vi "target.vi"   [LabVIEW 2020]
uses:
  <vilib>/rvi/interface/RandomDataEmulation/niFpgaRandomDataHandleErrors.vi
  <vilib>/rvi/DataTransferAndStorage/Container/XNode/niFpgaContainer.xnode
  <vilib>/rvi/interface/RandomDataEmulation/nirviRandomDataFpgaReadWriteTemplate.vi
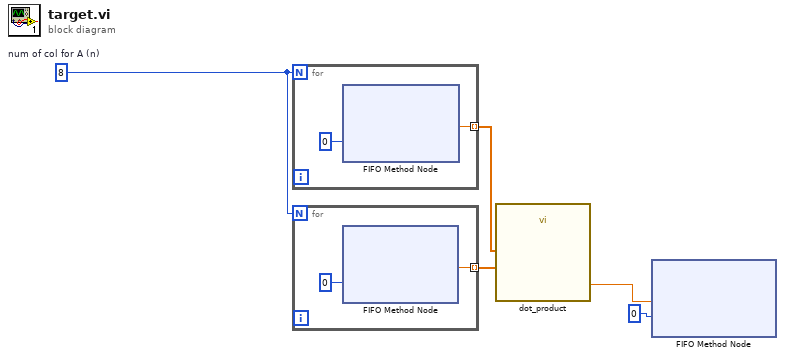
[diagram p0: block diagram]
diagram:
  w3 = 8  # num of col for A (n)
  n1 = for {
    N: w3 -> [_]
    tunnel: [w7] -> w5 mode=indexing
    n2 = xnode ("FIFO Method Node")("Timeout"=0) -> ("Element"=w7:sgl)  [unwired: 1 in, 2 out]
  }
  n3 = for {
    N: w3 -> [_]
    tunnel: [w8] -> w4 mode=indexing
    n4 = xnode ("FIFO Method Node")("Timeout"=0) -> ("Element"=w8:sgl)  [unwired: 1 in, 2 out]
  }
  n5 = call "dot_product.vi"("B"=w4, "A"=w5) -> ("c"=w2:sgl)
  n6 = xnode ("FIFO Method Node")("Element"=w2, "Timeout"=0) -> ()  [unwired: 1 in, 2 out]
